vi "Update Map - Safe Move.vi"(8 "Action Order":cluster{"Action":T2, "Direction":T1}[](array[cluster]), 9 "Column":i32, 10 "Row":i32, 11 "map in":refnum<data-value>) -> (0 "move accepted?":bool, 1 "Selected Direction":T1, 2 "Selected Action":T2, 3 "map out":refnum<data-value>)   [LabVIEW 2017, in "DS Square.lvlib"]
uses:
  DS Square.lvlib
  Map.ctl
  Square Status.ctl
  Square State.ctl
  Center of Mass.ctl
  Type Defs/Action Enum.ctl
  Type Defs/Direction Enum.ctl
  Common/Position.ctl
  Square/Board Size.vi
  SubVIs/Read-Only Globals.vi
  SubVIs/Globals (private).vi
  Common/Common.lvlib
  Type Defs/SB Type Defs.lvlib
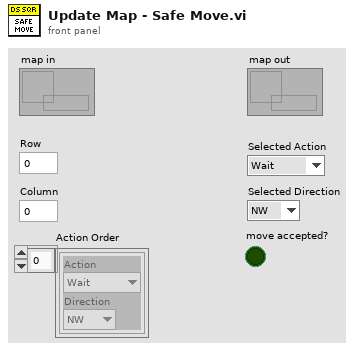
[diagram p1: front panel]
types:
  T1 = typedef "SB Type Defs.lvlib/Direction Enum.ctl" = enum16{"NW", "N", "NE", "E", "SE", "S", "SW", "W"}
  T2 = typedef "SB Type Defs.lvlib/Action Enum.ctl" = enum16{"Wait", "Move", "Attack", "Replicate"}
  T3 = typedef "Common.lvlib/Position.ctl" = cluster{"Column":i32, "Row":i32}
  T4 = typedef "DS Square.lvlib/Square State.ctl" = enum16{"Unknown", "Empty", "Occupied - Active", "Occupied - Cool Down", "Attacked", "Enemy", "Enemy Wall"}
  T5 = typedef "DS Square.lvlib/Map.ctl" = cluster{"squares":T6[][], "center of mass":T7}
  T6 = typedef "DS Square.lvlib/Square Status.ctl" = cluster{"square state":T4, "probability":dbl, "last update":i32}
  T7 = typedef "DS Square.lvlib/Center of Mass.ctl" = cluster{"row":dbl, "col":dbl, "mass":dbl}
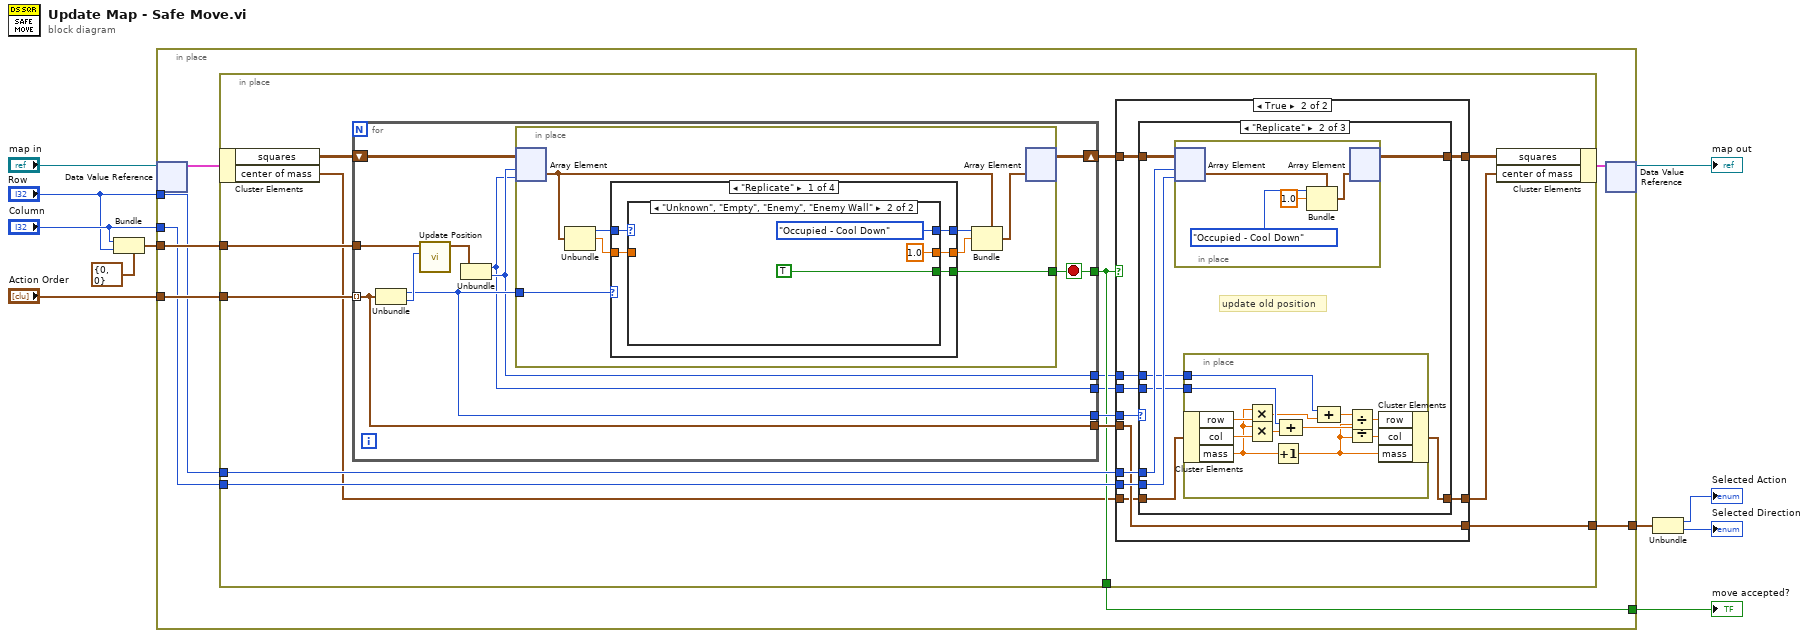
[diagram p0: block diagram]
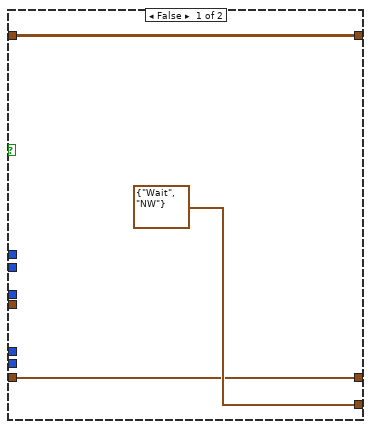
[diagram p2: hidden frame]
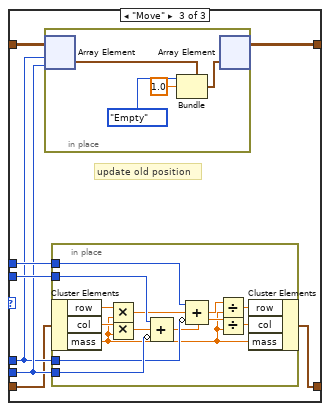
[diagram p4: hidden frame]
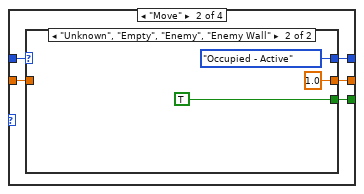
[diagram p6: hidden frame]
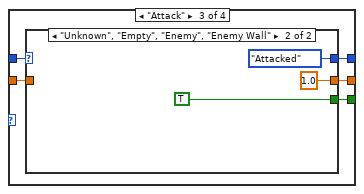
[diagram p8: hidden frame]
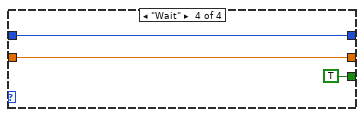
[diagram p10: hidden frame]
diagram:
  n1 = Bundle(cluster=T3 {"Column"=0, "Row"=0} ("Position in"), "Column"="Column", "Row"="Row") -> (w6:T3)
  n2 = in-place {
    in-place-border: "Row" -> [w17]
    in-place-border: "Column" -> [w16]
    in-place-border: w6 -> [w19]
    in-place-border: "Action Order" -> [w18]
    in-place-border: [w15] -> w4
    in-place-border: [w14] -> w1
    n3 = in-place-dvr #1("map in") -> (w13:T5)  [unwired: 1 out]
    n4 = in-place {
      in-place-border: w19 -> [w34]
      in-place-border: w18 -> [w33]
      in-place-border: w17 -> [w30]
      in-place-border: w16 -> [w29]
      in-place-border: [w27] -> w15
      in-place-border: [w26] -> w14
      n5 = in-place-cluster #2(w13) -> ("squares"=w25:T6[][], "center of mass"=w23:T7)
      n6 = for {
        tunnel: w34 -> [w108]
        shift-right: [w104] -> w32
        shift-left: w25 -> [w106]
        tunnel: w33 -> [w101] mode=indexing
        tunnel: [w103] -> w31
        tunnel: [w102] -> w26
        tunnel: [w101] -> w28
        tunnel: [w100] -> w22
        tunnel: [w99] -> w21
        stop <- w102 stop-if-true
        n7 = Unbundle(w101) -> ("Action"=w103:T2, "Direction"=w105:T1)
        n8 = call "Update Position.vi"("Direction"=w105, "Position in"=w108) -> ("Position out"=w107:T3)  [unwired: 9 in]
        n9 = Unbundle(w107) -> ("Column"=w99:i32, "Row"=w100:i32)
        n10 = in-place {
          in-place-border: [w113] -> w102
          in-place-border: w103 -> [w110]
          n11 = in-place-array #3(w106, w100, w99) -> (w115:T6)
          n12 = Unbundle(w115) -> ("square state"=w114:T4, "probability"=w112:dbl)  [unwired: 1 out]
          n13 = case shown="\"Replicate\"" w110 {
            tunnel: w114 -> [w121 w131 w141 w149]
            tunnel: [w120 w130 w140 w149] -> w109
            tunnel: [w119 w129 w139 TRUE] -> w113
            tunnel: w112 -> [w117 w127 w138 w148]
            tunnel: [w118 w128 w137 w148] -> w111
            frame "Replicate" {
              n14 = case shown="\"Unknown\", \"Empty\", \"Enemy\", \"Enemy Wall\"" w121 {
                selector: w121 -> [w123 _]
                tunnel: [w123 Square_State."Occupied - Cool Down" ("square state")] -> w120
                tunnel: [_ TRUE] -> w119
                tunnel: [w122 1.0 ("probability")] -> w118
                tunnel: w117 -> [w122 _]
                frame "Occupied - Active".."Attacked" {
                }
                frame "Unknown", "Empty", "Enemy", "Enemy Wall" {
                }
              }
            }
            frame "Move" {
              n15 = case shown="\"Unknown\", \"Empty\", \"Enemy\", \"Enemy Wall\"" w131 {
                selector: w131 -> [w133 _]
                tunnel: [w133 Square_State."Occupied - Active" ("square state")] -> w130
                tunnel: [_ TRUE] -> w129
                tunnel: [w132 1.0 ("probability")] -> w128
                tunnel: w127 -> [w132 _]
                frame "Occupied - Active".."Attacked" {
                }
                frame "Unknown", "Empty", "Enemy", "Enemy Wall" {
                }
              }
            }
            frame "Attack" {
              n16 = case shown="\"Unknown\", \"Empty\", \"Enemy\", \"Enemy Wall\"" w141 {
                selector: w141 -> [w143 _]
                tunnel: [w143 Square_State."Attacked" ("square state")] -> w140
                tunnel: [_ TRUE] -> w139
                tunnel: w138 -> [w142 _]
                tunnel: [w142 1.0 ("probability")] -> w137
                frame "Occupied - Active".."Attacked" {
                }
                frame "Unknown", "Empty", "Enemy", "Enemy Wall" {
                }
              }
            }
            frame "Wait" {
            }
          }
          n17 = Bundle(cluster=w115, "square state"=w109, "probability"=w111) -> (w116:T6)  [unwired: 1 in]
          n18 = in-place-array #3(w116) -> (w104:T6[][])  [unwired: 2 out]
        }
      }
      n19 = case shown="True" w26 {
        tunnel: w32 -> [w37 w47]
        tunnel: w31 -> [_ w46]
        tunnel: w30 -> [_ w45]
        tunnel: w29 -> [_ w44]
        tunnel: [w37 w43] -> w24
        tunnel: w28 -> [_ w42]
        tunnel: [cluster{"Action":T2, "Direction":T1} {"Action"=enum."Wait", "Direction"=enum."NW"} w42] -> w27
        tunnel: w23 -> [w35 w41]
        tunnel: w22 -> [_ w40]
        tunnel: w21 -> [_ w39]
        tunnel: [w35 w38] -> w20
        frame False {
        }
        frame True {
          n20 = case shown="\"Replicate\"" w46 {
            tunnel: w47 -> [w49 w57 w81]
            tunnel: w45 -> [_ w56 w76]
            tunnel: w44 -> [_ w55 w77]
            tunnel: [w49 w54 w80] -> w43
            tunnel: w41 -> [w48 w53 w75]
            tunnel: w40 -> [_ w51 w79]
            tunnel: w39 -> [_ w50 w78]
            tunnel: [w48 w52 w74] -> w38
            frame Default {
            }
            frame "Replicate" {
              # "update old position"
              n21 = in-place {
                n22 = in-place-array #4(w57, w56, w55) -> (w73:T6)
                n23 = Bundle(cluster=w73, "square state"=Square_State."Occupied - Cool Down", "probability"=1.0) -> (w72:T6)  [unwired: 1 in]
                n24 = in-place-array #4(w72) -> (w54:T6[][])  [unwired: 2 out]
              }
              n25 = in-place {
                in-place-border: w51 -> [w69]
                in-place-border: w50 -> [w68]
                n26 = in-place-cluster #5(w53) -> ("row"=w65:dbl, "col"=w66:dbl, "mass"=w64:dbl)
                n27 = Multiply(x=w64, y=w65) -> (x*y=w63:dbl)
                n28 = Multiply(x=w64, y=w66) -> (x*y=w67:dbl)
                n29 = Increment(x=w64) -> (x+1=w58:dbl)
                n30 = Compound Arithmetic op=ADD(w68, w67) -> (w61:dbl)
                n31 = Compound Arithmetic op=ADD(w69, w63) -> (w62:dbl)
                n32 = Divide(x=w62, y=w58) -> (x/y=w59:dbl)
                n33 = Divide(x=w61, y=w58) -> (x/y=w60:dbl)
                n34 = in-place-cluster #5("row"=w59, "col"=w60, "mass"=w58) -> (w52:T7)
              }
            }
            frame "Move" {
              # "update old position"
              n35 = in-place {
                n36 = in-place-array #6(w81, w76, w77) -> (w98:T6)
                n37 = Bundle(cluster=w98, "square state"=Square_State."Empty", "probability"=1.0) -> (w97:T6)  [unwired: 1 in]
                n38 = in-place-array #6(w97) -> (w80:T6[][])  [unwired: 2 out]
              }
              n39 = in-place {
                in-place-border: w79 -> [w94]
                in-place-border: w78 -> [w93]
                in-place-border: w77 -> [w92]
                in-place-border: w76 -> [w91]
                n40 = in-place-cluster #7(w75) -> ("row"=w89:dbl, "col"=w90:dbl, "mass"=w83:dbl)
                n41 = Multiply(x=w89, y=w83) -> (x*y=w87:dbl)
                n42 = Multiply(x=w90, y=w83) -> (x*y=w88:dbl)
                n43 = Compound Arithmetic op=ADD(w93, w88, invert w92) -> (w85:dbl)
                n44 = Compound Arithmetic op=ADD(w94, w87, invert w91) -> (w84:dbl)
                n45 = Divide(x=w84, y=w83) -> (x/y=w82:dbl)
                n46 = Divide(x=w85, y=w83) -> (x/y=w86:dbl)
                n47 = in-place-cluster #7("row"=w82, "col"=w86, "mass"=w83) -> (w74:T7)
              }
            }
          }
        }
      }
      n48 = in-place-cluster #2("squares"=w24, "center of mass"=w20) -> (w12:T5)
    }
    n49 = in-place-dvr #1(w12) -> (→"map out":refnum<data-value>)  [unwired: 1 out]
  }
  "move accepted?" <- w1
  n50 = Unbundle(w4) -> ("Action"=→"Selected Action":T2, "Direction"=→"Selected Direction":T1)
